vi "Do.vi"(8 "error in (no error)":errorcluster, 10 "Actor in":refnum<class "Actor.lvclass">, 11 "UpDataResult Msg":refnum<class "UpDataResult Msg.lvclass">) -> (0 "error out":errorcluster, 2 "Actor out":refnum<class "Actor.lvclass">)   [LabVIEW 2019, in "TestBench.lvlib" / "UpDataResult Msg.lvclass"]
doc: "This VI delivers the message to the actor by calling the appropriate method(s) on the actor."
uses:
  UpDataResult Msg.lvclass
  C:/Program Files (x86)/National Instruments/LabVIEW 2019/vi.lib/NI/Event Source Actor/Event Source/Event Source Messages/Event Generated Msg/Event Generated Msg.lvclass
  <vilib>/ActorFramework/Actor/Actor.lvclass
  TestBench/TestBench.lvclass
  C:/Program Files (x86)/National Instruments/LabVIEW 2019/vi.lib/ActorFramework/Actor/Actor.lvclass
  Assert/Assert/Assert Event.lvclass
  <vilib>/NI/Event Source Actor/Event Source/Event Source Messages/Event Generated Msg/Event Generated Msg.lvclass/Event Generated Msg.ctl
  <vilib>/NI/Event Source Actor/Event Source/Event Source Messages/Event Generated Msg/Event Generated Msg.lvclass
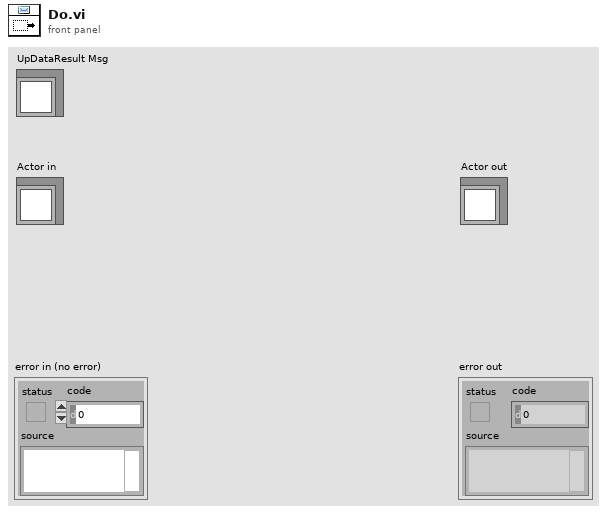
[diagram p1: front panel]
types:
  T1 = cluster{"UpDataResult":cluster{"Socket":i32, "Result":string, "Value":string, "Limit":cluster{"High":string, "Low":string}, "Type":string, "StepName":string, "Normal":string, "Unit":string}[], "Time":dbl}
  T2 = cluster{"Socket":i32, "Result":string, "Value":string, "Limit":cluster{"High":string, "Low":string}, "Type":string, "StepName":string, "Normal":string, "Unit":string}[]
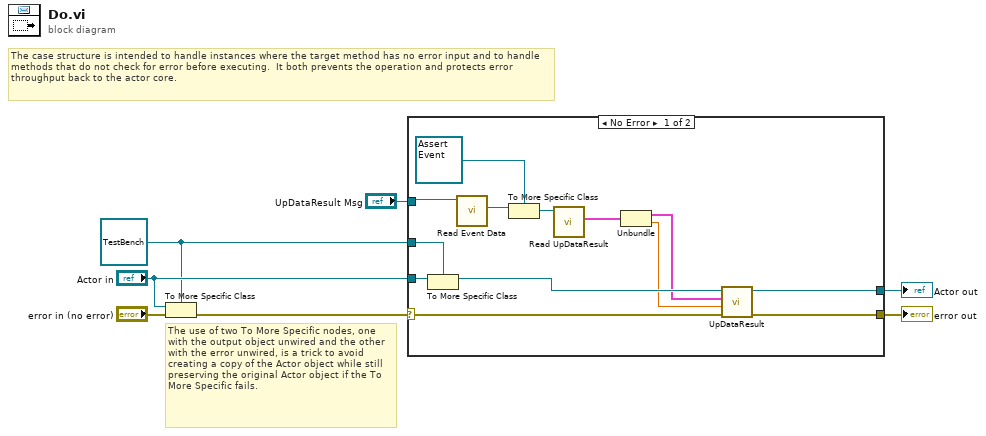
[diagram p0: block diagram]
diagram:
  w2 = refnum<class "TestBench.lvclass"> refnum ("Actor in")
  # "The use of two To More Specific nodes, one with the output object unwired and the other with the error unwired, is a trick to avoid creating a copy of the Actor object while still preserving the original Actor object if the To More Specific fails."
  # "The case structure is intended to handle instances where the target method has no error input and to handle methods that do not check for error before executing.  It both prevents the operation and protects error throughput back to the actor core."
  n1 = To More Specific Class(target class=w2, reference="Actor in", error in="error in (no error)") -> (error out=w6:errorcluster)  [unwired: 1 out]
  n2 = case shown="No Error" w6 {
    selector: w6 -> [w18 w22]
    tunnel: [w20 w22] -> w5
    tunnel: [w19 w21] -> w4
    tunnel: "Actor in" -> [w17 w21]
    tunnel: w2 -> [w16 _]
    tunnel: "UpDataResult Msg" -> [w12 _]
    frame No Error {
      n3 = To More Specific Class(target class=w16, reference=w17) -> (specific class reference=w15:refnum<class "TestBench.lvclass">)  [unwired: 1 in, 1 out]
      n4 = call <vilib>:"Read Event Data.vi"("Event Generated Msg"=w12) -> ("Event Data"=w14:refnum<class "Event.lvclass">)  [unwired: 10 in]
      n5 = To More Specific Class(target class=refnum<class "Assert Event.lvclass"> refnum ("Assert.lvlib:Assert Event.lvclass"), reference=w14) -> (specific class reference=w11:refnum<class "Assert Event.lvclass">)  [unwired: 1 in, 1 out]
      n6 = call-dynamic "Read UpDataResult.vi"("Assert Event in"=w11) -> ("UpDataResult"=w10:T1)  [unwired: 8 in, 2 out]
      n7 = Unbundle(w10) -> ("UpDataResult"=w9:T2, "Time"=w8:dbl)
      n8 = call-dynamic "UpDataResult.vi"("error in (no error)"=w18, "Time"=w8, "UpDataResult"=w9, "TestBench in"=w15) -> ("error out"=w20:errorcluster, "TestBench out"=w19:refnum<class "TestBench.lvclass">)  [unwired: 6 in]
    }
    frame Error {
      # "If type check fails, pass the original object out again."
    }
  }
  "error out" <- w5
  "Actor out" <- w4
